vi "Min Read Array.vi"(8 "error in":errorcluster, 11 "Min Current Limit in":refnum<class "Current Limit.lvclass">) -> (0 "error out":errorcluster, 1 "Changed or First Call?":bool, 2 "Current Min SP":dbl[](array[numeric]), 3 "Min Current Limit out":refnum<class "Current Limit.lvclass">)   [LabVIEW 2023, in "Current Limit.lvclass"]
uses:
  Current Limit.lvclass
  Parents/Limit/Limit.lvclass
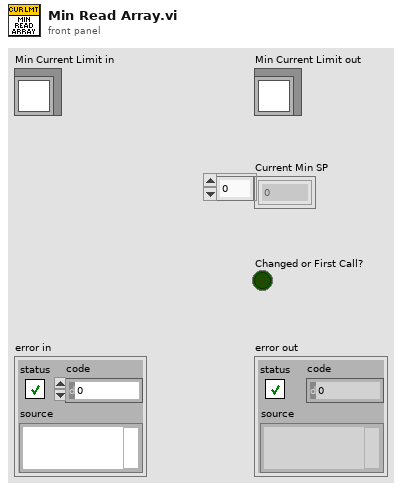
[diagram p1: front panel]
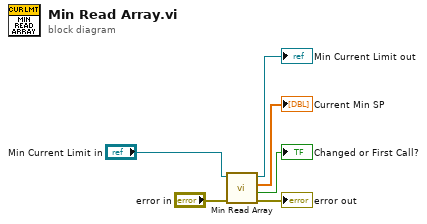
[diagram p0: block diagram]
diagram:
  n1 = call-parent "Min Read Array.vi"("error in"="error in", "Min Limit in"="Min Current Limit in") -> ("error out"=→"error out":errorcluster, "Changed or First Call?"=→"Changed or First Call?":bool, "Current Min SP"=→"Current Min SP":dbl[], "Min Limit out"=→"Min Current Limit out":refnum<class "Current Limit.lvclass">)  [unwired: 6 in]
